vi "Stop Point on Target.vi"(7 "Point Ident":string, 8 "error in":errorcluster, 11 "Study Actor in":refnum<class "Study Actor.lvclass">) -> (0 "error out":errorcluster, 3 "Study Actor out":refnum<class "Study Actor.lvclass">)   [LabVIEW 2023, in "Study Actor.lvlib" / "Study Actor.lvclass"]
uses:
  Study Actor.lvclass
  MSS Target/IMSS Target Actor Messages/Stop Point Msg/Stop Point Msg.lvclass/Stop Point Msg.ctl
  <vilib>/ActorFramework/Message Enqueuer/Message Enqueuer.lvclass/Message Enqueuer.ctl
  <vilib>/ActorFramework/Message Enqueuer/Enqueue.vi
  MSS Target/IMSS Target Actor Messages/Stop Point Msg/Stop Point Msg.lvclass
  <vilib>/Utility/LVClass/Get LV Class Name.vi
  <resource>/AFDebug/Generate Trace for Message.vi
  <vilib>/ActorFramework/Message Priority Queue/Priority Enqueue.vi
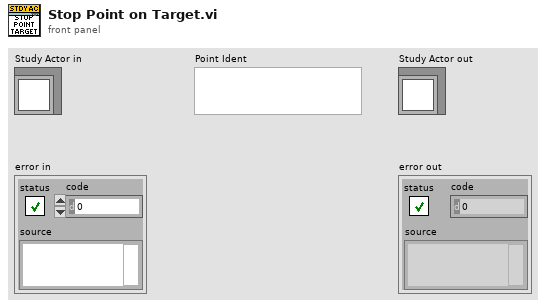
[diagram p1: front panel]
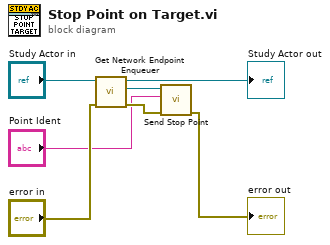
[diagram p0: block diagram]
diagram:
  n1 = call "Get Network Endpoint Enqueuer.vi"("error in"="error in", "Study Actor in"="Study Actor in") -> ("error out"=w3:errorcluster, "Network Endpoint Enqueuer"=w4:refnum<class "Message Enqueuer.lvclass">, "Study Actor out"=→"Study Actor out":refnum<class "Study Actor.lvclass">)  [unwired: 6 in, 1 out]
  n2 = call "Send Stop Point.vi"("error in (no error)"=w3, "Point Ident"="Point Ident", "Message Enqueuer"=w4) -> ("error out"=→"error out":errorcluster)  [unwired: 7 in, 1 out]
